vi "Reports_SoftwareStats.vi"(8 "Error In":errorcluster, 11 "All Team Software Data":string[][](array[string])) -> (0 "Error Out":errorcluster, 1 "Add-On SW Stats":cluster{"Add-On Types":string[], i32[][]}, 3 "Main SW Stats":cluster{string[], i32[][]})   [LabVIEW 2013, in "FIRST Reports.lvlib"]
uses:
  FIRST Reports.lvlib
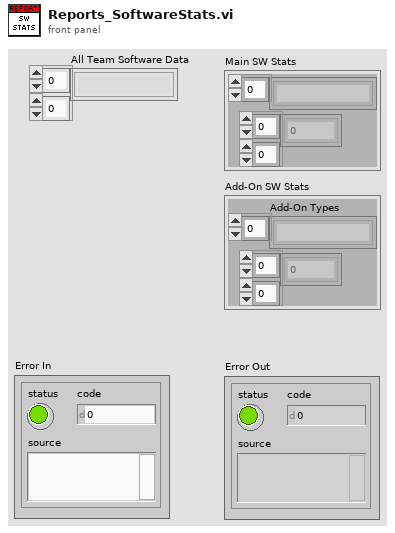
[diagram p1: front panel]
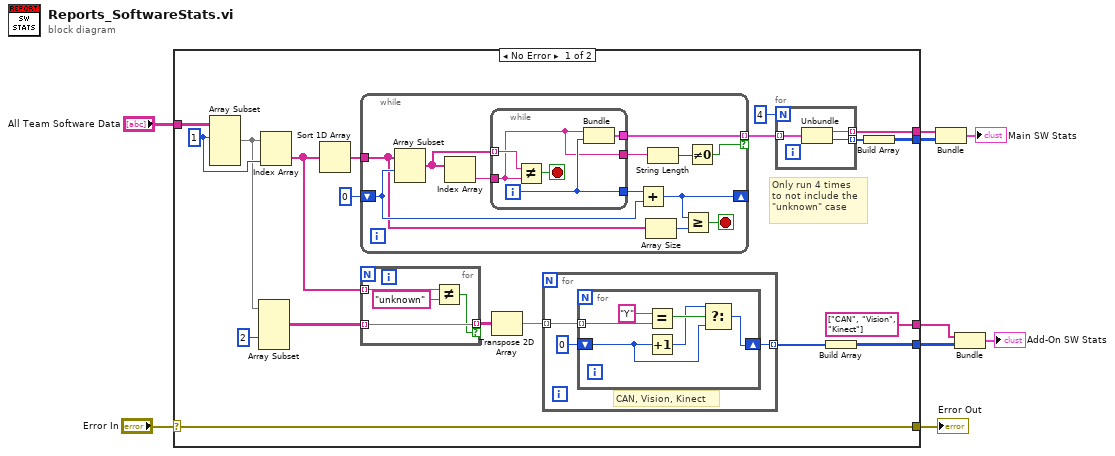
[diagram p0: block diagram]
diagram:
  n1 = case shown="No Error" "Error In" {
    selector: "Error In" -> [w22 w62]
    tunnel: [w26 _] -> w7
    tunnel: [w25 _] -> w6
    tunnel: "All Team Software Data" -> [w21 _]
    tunnel: [w22 w62] -> w8
    tunnel: [w11 _] -> w3
    tunnel: [string[] ["CAN", "Vision", "Kinect"] ("Add-On Types") _] -> w4
    frame No Error {
      w20 = 1 ("index")
      # "Only run 4 times \nto not include the\n\"unknown\" case"
      n2 = Array Subset(array=w21, index (row)=w20) -> (w19:string[][])  [unwired: 3 in]
      n3 = Array Subset(array=w19, index (col)=2 ("index")) -> (w15:string[][])  [unwired: 3 in]
      n4 = Index Array(array=w19, index (col)=w20) -> (element=w16:string[])  [unwired: 1 in]
      n5 = Sort 1D Array(array=w16) -> (sorted array=w17:string[])
      n6 = while {
        tunnel: [w55] -> w24 mode=indexing if=w46
        shift-right: [w51] -> _
        shift-left: 0 -> [w52]
        tunnel: w17 -> [w50]
        stop <- w48 stop-if-true
        n7 = Array Subset(array=w50, index=w52) -> (w54:string[])  [unwired: 1 in]
        n8 = Index Array(array=w54) -> (element=w56:string)  [unwired: 1 in]
        n9 = while {
          tunnel: w56 -> [w57]
          tunnel: w54 -> [w60] mode=indexing
          tunnel: [w59] -> w55
          tunnel: [w58] -> w53
          tunnel: [w57] -> w45
          i -> [w58]
          stop <- w61 stop-if-true
          n10 = Not Equal?(x=w60, y=w57) -> (x != y?=w61:bool)
          n11 = Bundle(w57, w58) -> (w59:cluster{string, i32})  [unwired: 1 in]
        }
        n12 = Add(x=w53, y=w52) -> (x+y=w51:i32)
        n13 = Array Size(array=w50) -> (size(s)=w49:i32)
        n14 = String Length(string=w45) -> (length=w47:i32)
        n15 = Greater Or Equal?(x=w51, y=w49) -> (x >= y?=w48:bool)
        n16 = Not Equal To 0?(x=w47) -> (x != 0?=w46:bool)
      }
      n17 = for {
        tunnel: w16 -> [w41] mode=indexing
        tunnel: w15 -> [w39] mode=indexing
        tunnel: [w39] -> w14 mode=indexing if=w38
        n18 = Not Equal?(x=w41, y="unknown") -> (x != y?=w38:bool)
      }
      n19 = Transpose 2D Array(2D array=w14) -> (transposed array=w13:string[][])
      n20 = for {
        tunnel: w13 -> [w31] mode=indexing
        tunnel: [w29] -> w12 mode=indexing
        # "CAN, Vision, Kinect"
        n21 = for {
          tunnel: w31 -> [w37] mode=indexing
          shift-right: [w35] -> w29
          shift-left: 0 -> [w32]
          n22 = Equal?(x="Y", y=w37) -> (x = y?=w34:bool)
          n23 = Increment(x=w32) -> (x+1=w33:i32)
          n24 = Select(t=w33, s=w34, f=w32) -> (s? t:f=w35:i32)
        }
      }
      n25 = for {
        N: 4 -> [_]
        tunnel: w24 -> [w44] mode=indexing
        tunnel: [w43] -> w25 mode=indexing
        tunnel: [w42] -> w27 mode=indexing
        n26 = Unbundle(w44) -> (w43:string, w42:i32)
      }
      n27 = Build Array(w12) -> (w11:i32[][])
      n28 = Build Array(w27) -> (w26:i32[][])
    }
    frame Error {
    }
  }
  "Error Out" <- w8
  n29 = Bundle(w6, w7) -> (→"Main SW Stats":cluster{string[], i32[][]})  [unwired: 1 in]
  n30 = Bundle("Add-On Types"=w4, w3) -> (→"Add-On SW Stats":cluster{"Add-On Types":string[], i32[][]})  [unwired: 1 in]
